vi "VariableValueToCluster.vi"(11 "VariableValue":refnum<class "VariableValue.lvclass">) -> (3 "VariableValueCluster":cluster{"Name":string, "Value":dbl})   [LabVIEW 2013, in "VariableManagerAPI.lvlib"]
uses:
  VariableManagerAPI.lvlib
  VariableValue/VariableValue.lvclass
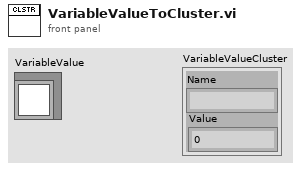
[diagram p1: front panel]
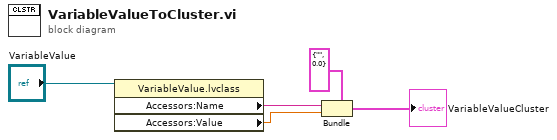
[diagram p0: block diagram]
diagram:
  n1 = property class="VariableValue.lvclass"(reference="VariableValue") -> ("Accessors:Name"=w4:string, "Accessors:Value"=w3:dbl)  [unwired: 1 in, 2 out]
  n2 = Bundle(cluster=cluster{"Name":string, "Value":dbl} {"Name"="", "Value"=0.0} ("VariableValueClusterOut 2"), "Name"=w4, "Value"=w3) -> (→"VariableValueCluster":cluster{"Name":string, "Value":dbl})
